vi "Calculate OUR.vi"(8 "error in (no error)":errorcluster, 11 "OUR_Monitor in":refnum<class "OUR_Monitor.lvclass">) -> (0 "error out":errorcluster, 3 "OUR_Monitor out":refnum<class "OUR_Monitor.lvclass">)   [LabVIEW 2021, in "MBPOnOff_Controller.lvlib" / "OUR_Monitor.lvclass"]
uses:
  OUR_Monitor.lvclass
  OUR_Monitor.lvclass/OUR_Monitor.ctl
  <vilib>/Analysis/NI_AALPro.lvlib
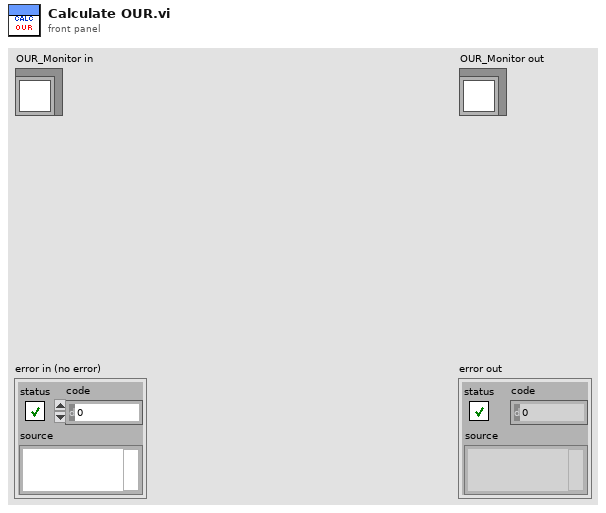
[diagram p1: front panel]
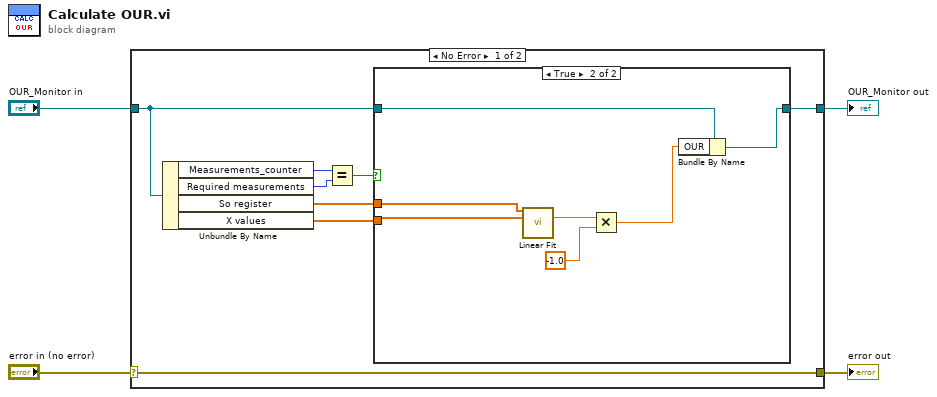
[diagram p0: block diagram]
diagram:
  n1 = case shown="No Error" "error in (no error)" {
    selector: "error in (no error)" -> [w12 w22]
    tunnel: [w12 w22] -> w3
    tunnel: [w10 w21] -> w1
    tunnel: "OUR_Monitor in" -> [w11 w21]
    frame No Error {
      n2 = Unbundle By Name(w11) -> ("Measurements_counter"=w9:i32, "Required measurements"=w8:i32, "So register"=w6:dbl[], "X values"=w5:dbl[])
      n3 = Equal?(x=w9, y=w8) -> (x = y?=w7:bool)
      n4 = case shown="True" w7 {
        tunnel: w11 -> [w13 w16]
        tunnel: [w13 w14] -> w10
        tunnel: w6 -> [_ w20]
        tunnel: w5 -> [_ w19]
        frame False {
        }
        frame True {
          n5 = call <vilib>:"Linear Fit.vi"("Y"=w20, "X"=w19) -> ("slope"=w17:dbl)  [unwired: 9 in, 4 out]
          n6 = Multiply(x=w17, y=-1.0) -> (x*y=w15:dbl)
          n7 = Bundle By Name(cluster=w16, "OUR"=w15) -> (w14:refnum<class "OUR_Monitor.lvclass">)
        }
      }
    }
    frame Error {
    }
  }
  "error out" <- w3
  "OUR_Monitor out" <- w1
